vi "openbci_new_cnx.vi"(6 "delay_tx (100ms)":u32=100, 7 "channel_count(8)":T3, 8 "error in (no error)":errorcluster, 9 "timeout (5sec)":u32=5000, 10 "baud rate (115200)":u32=115200, 11 "COM port":refnum<visa-resource-name>) -> (0 "error out":errorcluster, 3 "OBCI dev out":T2={"COM port"="", "n_ch (8)"=enum."8 Channels", "delay_tx"=50})   [LabVIEW 2013]
doc: "Serial Setup for OpenBCI V3\n\nDefault 115200bps 8-N-1\nTimeOut 5 seconds\nNumber of channels (8 Default)\nDelay between commands sent (50ms)"
uses:
  Control Def/channel_count.ctl
  Control Def/openbci_device.ctl
  <vilib>/Instr/_visa.llb/VISA Set IO Buffer Mask.ctl
  <vilib>/Instr/_visa.llb/VISA Configure Serial Port (Instr).vi
panel:
  in  "buffer size (32768)":u32=32768
  in  "Mask (48)":T1=48 items=["I/O Receive Buffer"=16, "I/O Transmit Buffer"=32, "I/O Receive and Transmit Buffer"=48]
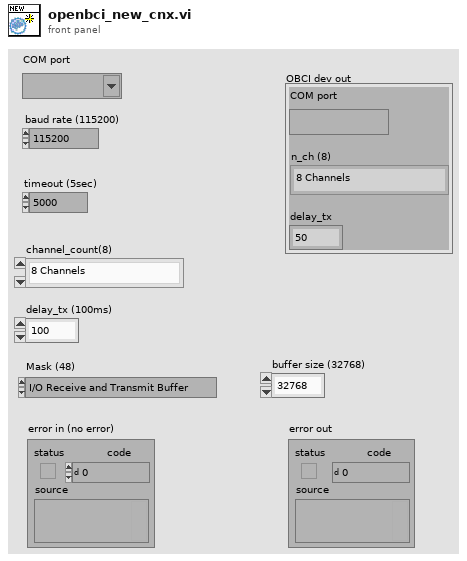
[diagram p1: front panel]
types:
  T1 = typedef "VISA Set IO Buffer Mask.ctl" = u16
  T2 = typedef "openbci_device.ctl" = cluster{"COM port":refnum<visa-resource-name>, "n_ch (8)":T3, "delay_tx":u32}
  T3 = typedef "channel_count.ctl" = enum16{"8 Channels", "16 Channels"}
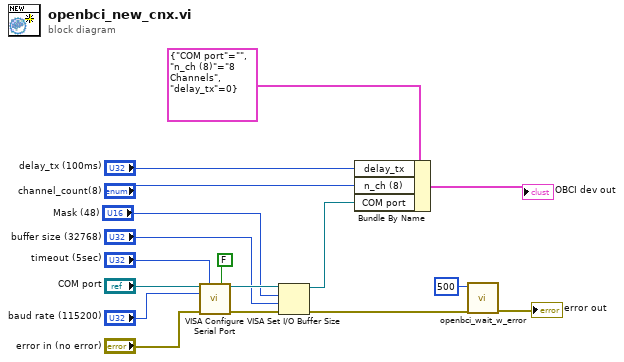
[diagram p0: block diagram]
diagram:
  n1 = call-poly "VISA Configure Serial Port"("VISA resource name"="COM port", "timeout (10sec)"="timeout (5sec)", "Enable Termination\nChar (T)"=FALSE ("Enable Termination\nChar (T)"), "baud rate (9600)"="baud rate (115200)", "error in (no error)"="error in (no error)") -> ("VISA resource name out"=w3:refnum<visa-resource-name>, "error out"=w6:errorcluster)  [unwired: 9 in]
  n2 = VISA Set I/O Buffer Size(VISA resource name=w3, mask (16)="Mask (48)", size (4096)="buffer size (32768)", error in (no error)=w6) -> (VISA resource name out=w4:refnum<visa-resource-name>, error out=w5:errorcluster)
  n3 = Bundle By Name(cluster=T2 {"COM port"="", "n_ch (8)"=enum."8 Channels", "delay_tx"=0} ("Cluster"), "delay_tx"="delay_tx (100ms)", "n_ch (8)"="channel_count(8)", "COM port"=w4) -> (→"OBCI dev out":T2)
  n4 = call "openbci_wait_w_error.vi"("error in (no error)"=w5, "milliseconds to wait"=u32 500) -> ("error out"=→"error out":errorcluster)  [unwired: 9 in]
